vi "Read AI.vi"(0 "FPGA AI Loop Data in":T1) -> (4 "FPGA AI Loop Data out":T1, 6 "Error AI mod 1":errorcluster, 8 "Error AI mod 2":errorcluster, 10 "FIFO AI Timed Out?":bool)   [LabVIEW 2019]
uses:
  TypeDef/FPGA AI Loop Data.ctl
  TypeDef/FPGA AIs.ctl
  <vilib>/rvi/eio/common/nirviEmuTemplateMethod_errors.vi
  <vilib>/rvi/interface/RandomDataEmulation/nirviRandomDataMultiElementFPGAFIFO.vi
  <instcachedir>/0/nirviRandomDataMultiElementFPGAFIFO_1ED88BA00AC641F388A9B1FAA20E354D.lvgen/nirviRandomDataMultiElementFPGAFIFO_1ED88BA00AC641F388A9B1FAA20E354D_004.vi
  <vilib>/rvi/interface/RandomDataEmulation/niFpgaRandomDataHandleErrors.vi
  <vilib>/eio/EIONode/EIONode.xnode
  <vilib>/rvi/Analysis/measure/notch/XNode/niFpgaNotchFilter.xnode
  <vilib>/rvi/Analysis/common/FxpNativeNode/niFpgaFxpNative.xnode
  <vilib>/rvi/DataTransferAndStorage/Container/XNode/niFpgaContainer.xnode
  <vilib>/rvi/interface/RandomDataEmulation/nirviRandomDataFpgaMultiElementTemplate.vi
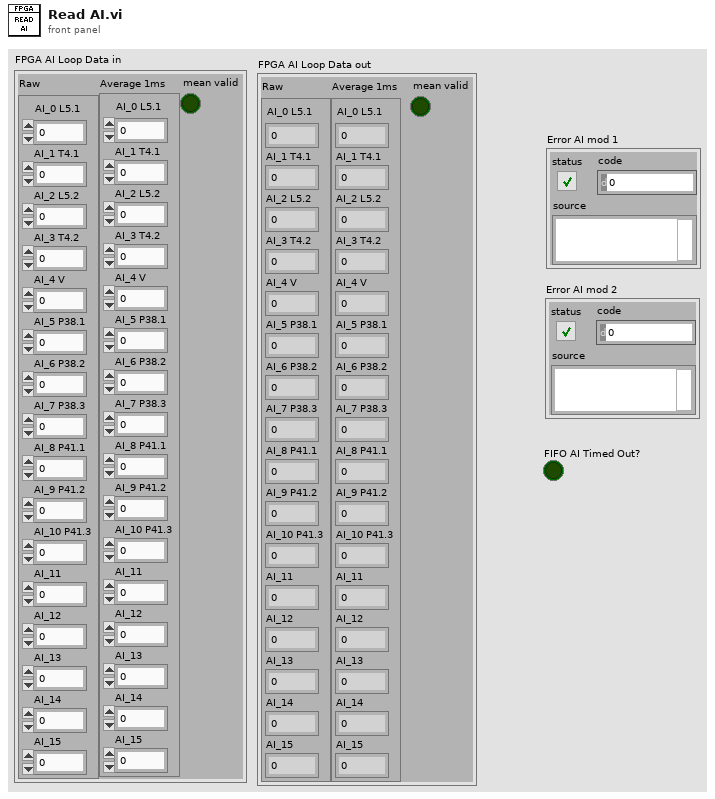
[diagram p1: front panel]
types:
  T1 = typedef "FPGA AI Loop Data.ctl" = cluster{"Raw":T2, "Average 1ms":T2, "mean valid":bool}
  T2 = typedef "FPGA AIs.ctl" = cluster{"AI_0 L5.1":fxp<+/-,21,-4>, "AI_1 T4.1":fxp<+/-,21,-4>, "AI_2 L5.2":fxp<+/-,21,-4>, "AI_3 T4.2":fxp<+/-,21,-4>, "AI_4 V":fxp<+/-,21,-4>, "AI_5 P38.1":fxp<+/-,21,-4>, "AI_6 P38.2":fxp<+/-,21,-4>, "AI_7 P38.3":fxp<+/-,21,-4>, "AI_8 P41.1":fxp<+/-,21,-4>, "AI_9 P41.2":fxp<+/-,21,-4>, "AI_10 P41.3":fxp<+/-,21,-4>, "AI_11":fxp<+/-,21,-4>, "AI_12":fxp<+/-,21,-4>, "AI_13":fxp<+/-,21,-4>, "AI_14":fxp<+/-,21,-4>, "AI_15":fxp<+/-,21,-4>}
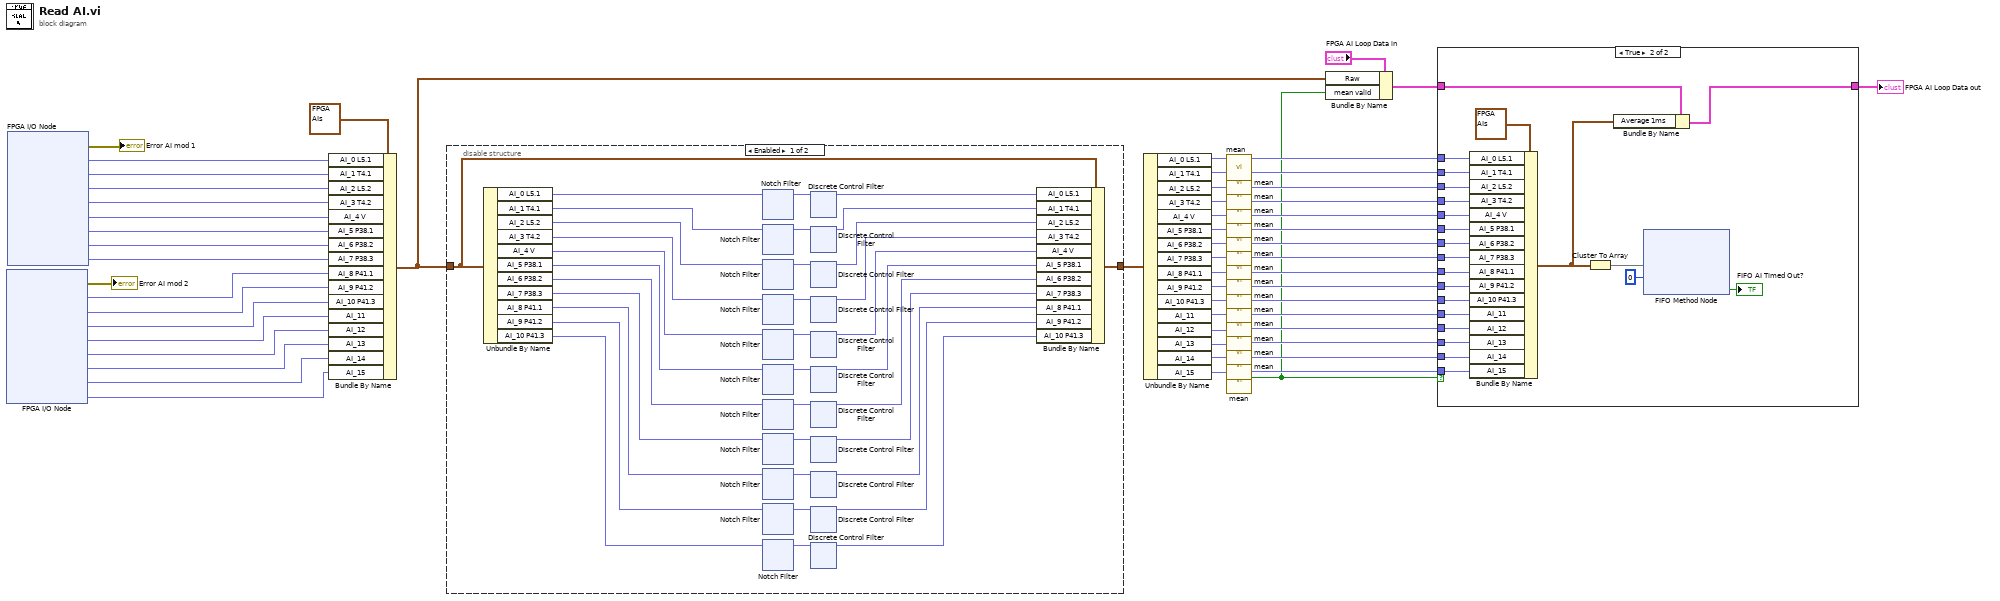
[diagram p0: block diagram]
diagram:
  n1 = xnode "FPGA I/O Node"() -> ("error out"=→"Error AI mod 2":errorcluster, "Mod4/AI0"=w46:fxp<+/-,21,-4>, "Mod4/AI1"=w45:fxp<+/-,21,-4>, "Mod4/AI2"=w44:fxp<+/-,21,-4>, "Mod4/AI3"=w19:fxp<+/-,21,-4>, "Mod4/AI4"=w18:fxp<+/-,21,-4>, "Mod4/AI5"=w17:fxp<+/-,21,-4>, "Mod4/AI6"=w16:fxp<+/-,21,-4>, "Mod4/AI7"=w15:fxp<+/-,21,-4>)  [unwired: 9 in, 8 out]
  n2 = xnode "FPGA I/O Node"() -> ("error out"=→"Error AI mod 1":errorcluster, "Mod3/AI0"=w54:fxp<+/-,21,-4>, "Mod3/AI1"=w53:fxp<+/-,21,-4>, "Mod3/AI2"=w52:fxp<+/-,21,-4>, "Mod3/AI3"=w51:fxp<+/-,21,-4>, "Mod3/AI4"=w50:fxp<+/-,21,-4>, "Mod3/AI5"=w49:fxp<+/-,21,-4>, "Mod3/AI6"=w48:fxp<+/-,21,-4>, "Mod3/AI7"=w47:fxp<+/-,21,-4>)  [unwired: 9 in, 8 out]
  n3 = Bundle By Name(cluster=T2 {"AI_0 L5.1"=0.0, "AI_1 T4.1"=0.0, "AI_2 L5.2"=0.0, "AI_3 T4.2"=0.0, "AI_4 V"=0.0, "AI_5 P38.1"=0.0, "AI_6 P38.2"=0.0, "AI_7 P38.3"=0.0, "AI_8 P41.1"=0.0, "AI_9 P41.2"=0.0, "AI_10 P41.3"=0.0, "AI_11"=0.0, "AI_12"=0.0, "AI_13"=0.0, "AI_14"=0.0, "AI_15"=0.0} ("FPGA AIs"), "AI_0 L5.1"=w54, "AI_1 T4.1"=w53, "AI_2 L5.2"=w52, "AI_3 T4.2"=w51, "AI_4 V"=w50, "AI_5 P38.1"=w49, "AI_6 P38.2"=w48, "AI_7 P38.3"=w47, "AI_8 P41.1"=w46, "AI_9 P41.2"=w45, "AI_10 P41.3"=w44, "AI_11"=w19, "AI_12"=w18, "AI_13"=w17, "AI_14"=w16, "AI_15"=w15) -> (w4:T2)
  n4 = disable-structure shown="Enabled" {
    disable-tunnel: [w92 _] -> w2
    disable-tunnel: w4 -> [w80 _]
    frame Enabled {
      n5 = Unbundle By Name(w80) -> ("AI_0 L5.1"=w69:fxp<+/-,21,-4>, "AI_1 T4.1"=w70:fxp<+/-,21,-4>, "AI_2 L5.2"=w71:fxp<+/-,21,-4>, "AI_3 T4.2"=w72:fxp<+/-,21,-4>, "AI_4 V"=w73:fxp<+/-,21,-4>, "AI_5 P38.1"=w74:fxp<+/-,21,-4>, "AI_6 P38.2"=w75:fxp<+/-,21,-4>, "AI_7 P38.3"=w76:fxp<+/-,21,-4>, "AI_8 P41.1"=w77:fxp<+/-,21,-4>, "AI_9 P41.2"=w78:fxp<+/-,21,-4>, "AI_10 P41.3"=w79:fxp<+/-,21,-4>)
      n6 = xnode "Notch Filter"("input data"=w69) -> ("output data"=w68:fxp<+/-,21,-4>)  [unwired: 2 in]
      n7 = xnode "Notch Filter"("input data"=w70) -> ("output data"=w67:fxp<+/-,21,-4>)  [unwired: 2 in]
      n8 = xnode "Notch Filter"("input data"=w71) -> ("output data"=w66:fxp<+/-,21,-4>)  [unwired: 2 in]
      n9 = xnode "Notch Filter"("input data"=w72) -> ("output data"=w64:fxp<+/-,21,-4>)  [unwired: 2 in]
      n10 = xnode "Notch Filter"("input data"=w73) -> ("output data"=w63:fxp<+/-,21,-4>)  [unwired: 2 in]
      n11 = xnode "Notch Filter"("input data"=w74) -> ("output data"=w62:fxp<+/-,21,-4>)  [unwired: 2 in]
      n12 = xnode "Notch Filter"("input data"=w75) -> ("output data"=w61:fxp<+/-,21,-4>)  [unwired: 2 in]
      n13 = xnode "Notch Filter"("input data"=w76) -> ("output data"=w60:fxp<+/-,21,-4>)  [unwired: 2 in]
      n14 = xnode "Notch Filter"("input data"=w77) -> ("output data"=w59:fxp<+/-,21,-4>)  [unwired: 2 in]
      n15 = xnode "Notch Filter"("input data"=w78) -> ("output data"=w58:fxp<+/-,21,-4>)  [unwired: 2 in]
      n16 = xnode "Notch Filter"("input data"=w79) -> ("output data"=w65:fxp<+/-,21,-4>)  [unwired: 2 in]
      n17 = xnode ("Discrete Control Filter")("input"=w68) -> ("output"=w91:fxp<+/-,21,-4>)  [unwired: 1 in]
      n18 = xnode ("Discrete Control Filter")("input"=w67) -> ("output"=w90:fxp<+/-,21,-4>)  [unwired: 1 in]
      n19 = xnode ("Discrete Control Filter")("input"=w66) -> ("output"=w89:fxp<+/-,21,-4>)  [unwired: 1 in]
      n20 = xnode ("Discrete Control Filter")("input"=w64) -> ("output"=w88:fxp<+/-,21,-4>)  [unwired: 1 in]
      n21 = xnode ("Discrete Control Filter")("input"=w63) -> ("output"=w87:fxp<+/-,21,-4>)  [unwired: 1 in]
      n22 = xnode ("Discrete Control Filter")("input"=w62) -> ("output"=w86:fxp<+/-,21,-4>)  [unwired: 1 in]
      n23 = xnode ("Discrete Control Filter")("input"=w61) -> ("output"=w85:fxp<+/-,21,-4>)  [unwired: 1 in]
      n24 = xnode ("Discrete Control Filter")("input"=w60) -> ("output"=w84:fxp<+/-,21,-4>)  [unwired: 1 in]
      n25 = xnode ("Discrete Control Filter")("input"=w59) -> ("output"=w83:fxp<+/-,21,-4>)  [unwired: 1 in]
      n26 = xnode ("Discrete Control Filter")("input"=w58) -> ("output"=w82:fxp<+/-,21,-4>)  [unwired: 1 in]
      n27 = xnode ("Discrete Control Filter")("input"=w65) -> ("output"=w81:fxp<+/-,21,-4>)  [unwired: 1 in]
      n28 = Bundle By Name(cluster=w80, "AI_0 L5.1"=w91, "AI_1 T4.1"=w90, "AI_2 L5.2"=w89, "AI_3 T4.2"=w88, "AI_4 V"=w87, "AI_5 P38.1"=w86, "AI_6 P38.2"=w85, "AI_7 P38.3"=w84, "AI_8 P41.1"=w83, "AI_9 P41.2"=w82, "AI_10 P41.3"=w81) -> (w92:T2)
    }
    frame Disabled {
    }
  }
  n29 = Unbundle By Name(w2) -> ("AI_0 L5.1"=w43:fxp<+/-,21,-4>, "AI_1 T4.1"=w42:fxp<+/-,21,-4>, "AI_2 L5.2"=w41:fxp<+/-,21,-4>, "AI_3 T4.2"=w40:fxp<+/-,21,-4>, "AI_4 V"=w39:fxp<+/-,21,-4>, "AI_5 P38.1"=w38:fxp<+/-,21,-4>, "AI_6 P38.2"=w37:fxp<+/-,21,-4>, "AI_7 P38.3"=w36:fxp<+/-,21,-4>, "AI_8 P41.1"=w35:fxp<+/-,21,-4>, "AI_9 P41.2"=w34:fxp<+/-,21,-4>, "AI_10 P41.3"=w33:fxp<+/-,21,-4>, "AI_11"=w14:fxp<+/-,21,-4>, "AI_12"=w13:fxp<+/-,21,-4>, "AI_13"=w12:fxp<+/-,21,-4>, "AI_14"=w11:fxp<+/-,21,-4>, "AI_15"=w10:fxp<+/-,21,-4>)
  n30 = call "mean.vi"("in"=w43) -> ("out"=w32:fxp<+/-,21,-4>)  [unwired: 9 in, 1 out]
  n31 = call "mean.vi"("in"=w42) -> ("out"=w31:fxp<+/-,21,-4>)  [unwired: 9 in, 1 out]
  n32 = call "mean.vi"("in"=w41) -> ("out"=w30:fxp<+/-,21,-4>)  [unwired: 9 in, 1 out]
  n33 = call "mean.vi"("in"=w40) -> ("out"=w29:fxp<+/-,21,-4>)  [unwired: 9 in, 1 out]
  n34 = call "mean.vi"("in"=w39) -> ("out"=w28:fxp<+/-,21,-4>)  [unwired: 9 in, 1 out]
  n35 = call "mean.vi"("in"=w38) -> ("out"=w27:fxp<+/-,21,-4>)  [unwired: 9 in, 1 out]
  n36 = call "mean.vi"("in"=w37) -> ("out"=w26:fxp<+/-,21,-4>)  [unwired: 9 in, 1 out]
  n37 = call "mean.vi"("in"=w36) -> ("out"=w25:fxp<+/-,21,-4>)  [unwired: 9 in, 1 out]
  n38 = call "mean.vi"("in"=w35) -> ("out"=w24:fxp<+/-,21,-4>)  [unwired: 9 in, 1 out]
  n39 = call "mean.vi"("in"=w34) -> ("out"=w23:fxp<+/-,21,-4>)  [unwired: 9 in, 1 out]
  n40 = call "mean.vi"("in"=w33) -> ("out"=w22:fxp<+/-,21,-4>)  [unwired: 9 in, 1 out]
  n41 = call "mean.vi"("in"=w14) -> ("out"=w5:fxp<+/-,21,-4>)  [unwired: 9 in, 1 out]
  n42 = call "mean.vi"("in"=w13) -> ("out"=w6:fxp<+/-,21,-4>)  [unwired: 9 in, 1 out]
  n43 = call "mean.vi"("in"=w12) -> ("out"=w7:fxp<+/-,21,-4>)  [unwired: 9 in, 1 out]
  n44 = call "mean.vi"("in"=w11) -> ("out"=w8:fxp<+/-,21,-4>)  [unwired: 9 in, 1 out]
  n45 = call "mean.vi"("in"=w10) -> ("output valid"=w3:bool, "out"=w9:fxp<+/-,21,-4>)  [unwired: 9 in]
  n46 = Bundle By Name(cluster="FPGA AI Loop Data in", "Raw"=w4, "mean valid"=w3) -> (w20:T1)
  n47 = case shown="True" w3 {
    tunnel: w32 -> [_ w544]
    tunnel: w31 -> [_ w543]
    tunnel: w30 -> [_ w542]
    tunnel: w29 -> [_ w541]
    tunnel: w28 -> [_ w540]
    tunnel: w27 -> [_ w539]
    tunnel: w26 -> [_ w538]
    tunnel: w25 -> [_ w537]
    tunnel: w24 -> [_ w536]
    tunnel: w23 -> [_ w535]
    tunnel: w22 -> [_ w534]
    tunnel: w20 -> [w522 w533]
    tunnel: w9 -> [_ w532]
    tunnel: w8 -> [_ w531]
    tunnel: w7 -> [_ w530]
    tunnel: w6 -> [_ w529]
    tunnel: w5 -> [_ w528]
    tunnel: [w522 w527] -> w1
    frame False {
    }
    frame True {
      n48 = Bundle By Name(cluster=T2 {"AI_0 L5.1"=0.0, "AI_1 T4.1"=0.0, "AI_2 L5.2"=0.0, "AI_3 T4.2"=0.0, "AI_4 V"=0.0, "AI_5 P38.1"=0.0, "AI_6 P38.2"=0.0, "AI_7 P38.3"=0.0, "AI_8 P41.1"=0.0, "AI_9 P41.2"=0.0, "AI_10 P41.3"=0.0, "AI_11"=0.0, "AI_12"=0.0, "AI_13"=0.0, "AI_14"=0.0, "AI_15"=0.0} ("FPGA AIs"), "AI_0 L5.1"=w544, "AI_1 T4.1"=w543, "AI_2 L5.2"=w542, "AI_3 T4.2"=w541, "AI_4 V"=w540, "AI_5 P38.1"=w539, "AI_6 P38.2"=w538, "AI_7 P38.3"=w537, "AI_8 P41.1"=w536, "AI_9 P41.2"=w535, "AI_10 P41.3"=w534, "AI_11"=w528, "AI_12"=w529, "AI_13"=w530, "AI_14"=w531, "AI_15"=w532) -> (w526:T2)
      n49 = Cluster To Array(cluster=w526) -> (array=w525:fxp<+/-,21,-4>[])
      n50 = Bundle By Name(cluster=w533, "Average 1ms"=w526) -> (w527:T1)
      n51 = xnode ("FIFO Method Node")("Element"=w525, "Timeout"=0) -> ("Timed Out?"=→"FIFO AI Timed Out?":bool)  [unwired: 1 in, 1 out]
    }
  }
  "FPGA AI Loop Data out" <- w1
